vi "Wavelength Digikröm.vi"(8 "error in (no error)":errorcluster, 10 "Spectrometer Digikröm.lvclass":refnum<class "Spectrometer Digikröm.lvclass">, 11 "Wavelength Digikröm in":refnum<class "Wavelength Digikröm.lvclass">) -> (0 "error out":errorcluster, 3 "Wavelength Digikröm out":refnum<class "Wavelength Digikröm.lvclass">)   [LabVIEW 2009, in "Wavelength Digikröm.lvclass"]
uses:
  Wavelength Digikröm.lvclass
  Instruments/Spectrometer Digikröm/Spectrometer Digikröm.lvclass
  Global/GPIB Numbers.vi
  Wavelength Digikröm.lvclass/Wavelength Digikröm.ctl
  Scanner/Scanner.lvclass
  Instruments/Spectrometer Digikröm/Digikrom DK24x/Digikrom DK24x.lvlib
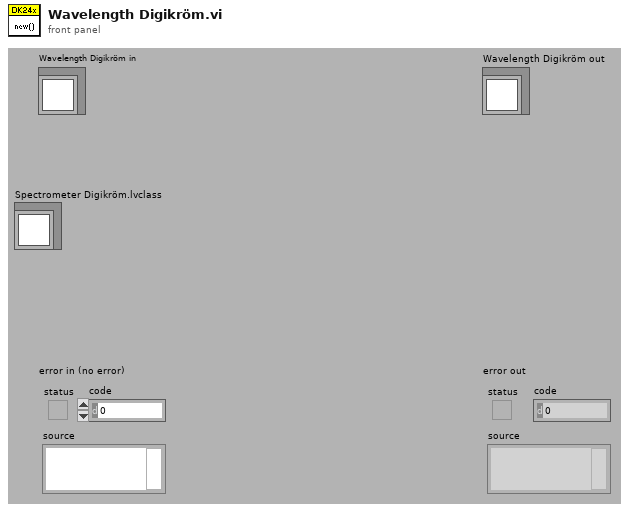
[diagram p1: front panel]
types:
  T1 = typedef "GPIB Type Def.ctl" = cluster{"Name":string, "bus":dbl, "GPIB":dbl, "GPIB as string":string, "byte":i32, "VISA Resource Name":refnum<visa-resource-name>}
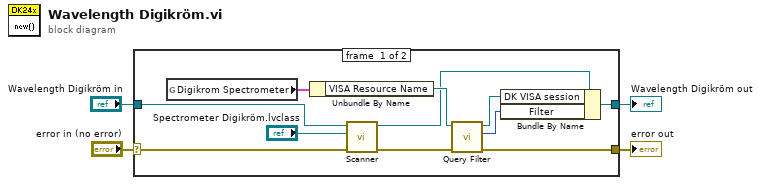
[diagram p0: block diagram]
diagram:
  n1 = case shown="No Error" "error in (no error)" {
    selector: "error in (no error)" -> [w14 w17]
    tunnel: [w11 w17] -> w3
    tunnel: [w5 w16] -> w1
    tunnel: "Wavelength Digikröm in" -> [w15 w16]
    frame #0 {
      n2 = global read "GPIB Numbers.vi" "Digikrom Spectrometer"() -> (w10:T1)
      n3 = Unbundle By Name(w10) -> ("VISA Resource Name"=w9:refnum<visa-resource-name>)
      n4 = call "Scanner.vi"("error in (no error)"=w14, "Scannable"="Spectrometer Digikröm.lvclass", "Scanner.lvclass in"=w15) -> ("error out"=w12:errorcluster, "Scanner.lvclass out"=w8:refnum<class "Wavelength Digikröm.lvclass">)  [unwired: 1 in, 6 out]
      n5 = call "Query Filter.vi"("error in (no error)"=w12, "VISA resource name"=w9) -> ("error out"=w11:errorcluster, "CURRENT FILTER"=w6:u8, "VISA resource name out"=w7:refnum<visa-resource-name>)  [unwired: 7 in]
      n6 = Bundle By Name(cluster=w8, "DK VISA session"=w7, "Filter"=w6) -> (w5:refnum<class "Wavelength Digikröm.lvclass">)
    }
    frame #1 {
    }
  }
  "error out" <- w3
  "Wavelength Digikröm out" <- w1
